vi "fgt get absolute Pressure Range.vi"(8 "error in (no error)":errorcluster, 11 "sensorIndex":u32) -> (0 "error out":errorcluster, 2 "pmax":sgl, 3 "pmin":sgl)   [LabVIEW 2016, in "fgt_SDK.lvlib"]
doc: "Returns the range of the absolute pressure sensor in mbar. This feature is only available on NIFS devices."
uses:
  fgt_SDK.lvlib
  dlls/fgt_SDK_32.dll
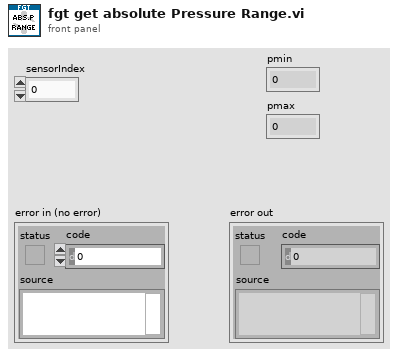
[diagram p1: front panel]
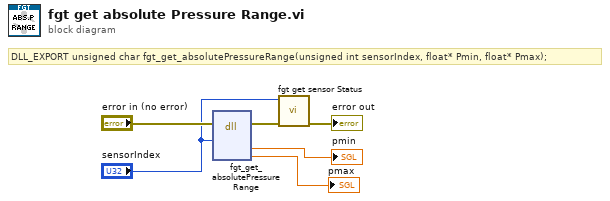
[diagram p0: block diagram]
diagram:
  # "DLL_EXPORT unsigned char fgt_get_absolutePressureRange(unsigned int sensorIndex, float* Pmin, float* Pmax);"
  n1 = dll-call lib="C:/projects/SDK/fgt-sdk-labview/dlls/fgt_SDK_*.*" fn="fgt_get_absolutePressureRange"(error in="error in (no error)", "sensorIndex"="sensorIndex") -> (error out=w4:errorcluster, "pmin"=→"pmin":sgl, "pmax"=→"pmax":sgl)  [unwired: 6 in, 1 out]
  n2 = call "fgt get sensor Status.vi"("error in (no error)"=w4, "pressureIndex"="sensorIndex") -> ("error out"=→"error out":errorcluster)  [unwired: 9 in]
